vi "ExternalVIDefaultLoad.vi"(11 "VI in":refnum<vi>) -> (3 "Update?":bool)   [LabVIEW 2020]
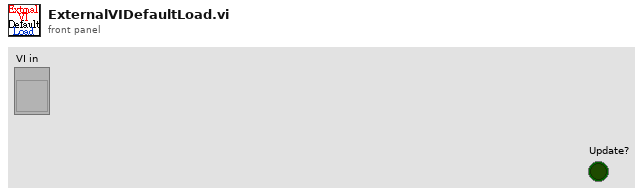
[diagram p1: front panel]
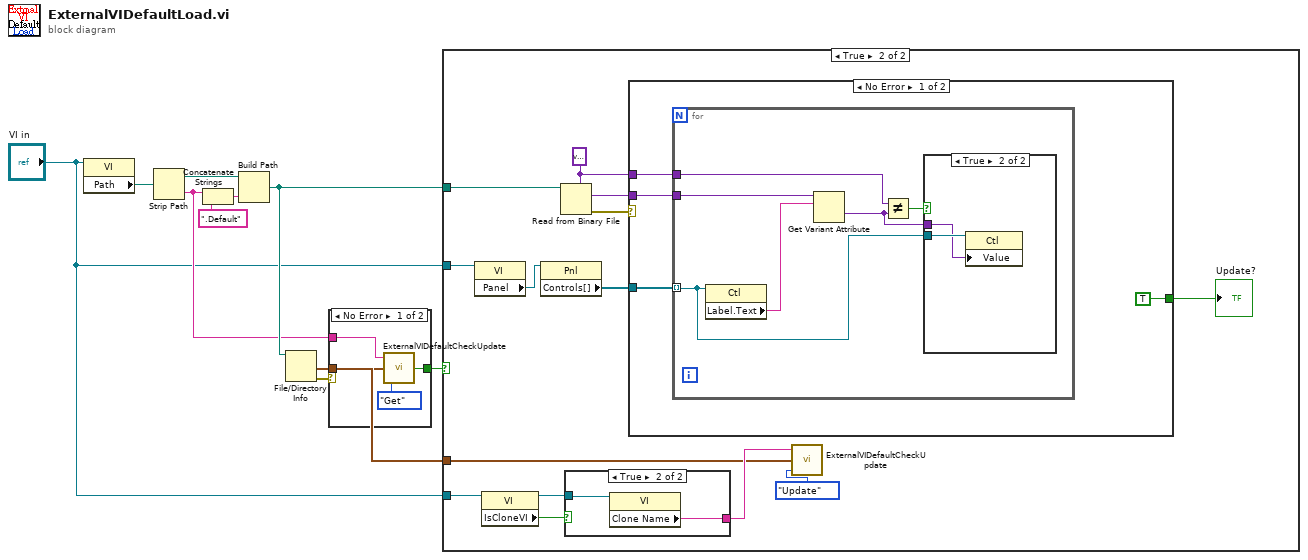
[diagram p0: block diagram]
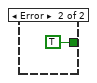
[diagram p2: hidden frame]
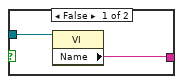
[diagram p4: hidden frame]
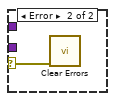
[diagram p6: hidden frame]
diagram:
  n1 = property class="VI"(reference="VI in") -> ("Path"=w7:path)  [unwired: 1 in, 2 out]
  n2 = Strip Path(path=w7) -> (stripped path=w9:path, name=w5:string)
  n3 = Concatenate Strings(w5, ".Default" ("string")) -> (w10:string)
  n4 = Build Path(base path=w9, name or relative path=w10) -> (appended path=w6:path)
  n5 = File/Directory Info(path=w6) -> (last mod=w3:timestamp, error out=w1:errorcluster)  [unwired: 1 in, 5 out]
  n6 = case shown="No Error" w1 {
    tunnel: w5 -> [w14 _]
    tunnel: [w12 TRUE ("NeedUpdate?")] -> w4
    tunnel: w3 -> [w11 _]
    frame No Error {
      n7 = call "ExternalVIDefaultCheckUpdate.vi"("OP"=enum16{"Get", "Update", "Init"}."Get", "last mod"=w11, "VIName"=w14) -> ("NeedUpdate?"=w12:bool)  [unwired: 1 in, 1 out]
    }
    frame Error {
    }
  }
  n8 = case shown="True" w4 {
    tunnel: "VI in" -> [_ w29]
    tunnel: w6 -> [_ w22]
    tunnel: w3 -> [_ w16]
    tunnel: "VI in" -> [_ w20]
    frame False {
    }
    frame True {
      w25 = variant
      n9 = property class="VI"(reference=w29) -> ("Panel"=w28:refnum<vi>)  [unwired: 1 in, 2 out]
      n10 = property class="VI"(reference=w20) -> (reference out=w18:refnum<vi>, "IsCloneVI"=w19:bool)  [unwired: 1 in, 1 out]
      n11 = property class="Pnl"(reference=w28) -> ("Controls[]"=w26:refnum<vi>[])  [unwired: 1 in, 2 out]
      n12 = Read from Binary File(5:w25, 11:w22) -> (0:w24:errorcluster, 2:w27:variant)  [unwired: 4 in, 2 out]
      n13 = case shown="True" w19 {
        tunnel: w18 -> [w31 w33]
        tunnel: [w30 w32] -> w17
        frame False {
          n14 = property class="VI"(reference=w31) -> ("Name"=w30:string)  [unwired: 1 in, 2 out]
        }
        frame True {
          n15 = property class="VI"(reference=w33) -> ("Clone Name"=w32:string)  [unwired: 1 in, 2 out]
        }
      }
      n16 = case shown="No Error" w24 {
        selector: w24 -> [_ w46]
        tunnel: w27 -> [w37 _]
        tunnel: w26 -> [w36 _]
        tunnel: w25 -> [w35 _]
        tunnel: [TRUE _] -> w23
        frame No Error {
          n17 = for {
            tunnel: w37 -> [w43]
            tunnel: w36 -> [w40] mode=indexing
            tunnel: w35 -> [w38]
            n18 = property class="Ctl"(reference=w40) -> ("Label.Text"=w42:string)  [unwired: 1 in, 2 out]
            n19 = Get Variant Attribute(Variant=w43, name=w42) -> (value=w39:variant)  [unwired: 2 in, 3 out]
            n20 = Not Equal?(x=w38, y=w39) -> (x != y?=w41:bool)
            n21 = case shown="True" w41 {
              tunnel: w40 -> [_ w45]
              tunnel: w39 -> [_ w44]
              frame False {
              }
              frame True {
                n22 = property class="Ctl"(reference=w45, "Value"=w44) -> ()  [unwired: 1 in, 2 out]
              }
            }
          }
        }
        frame Error {
          n23 = call <vilib>:"Clear Errors.vi"("error in (no error)"=w46) -> ()  [unwired: 5 in, 2 out]
        }
      }
      "Update?" <- w23
      n24 = call "ExternalVIDefaultCheckUpdate.vi"("OP"=enum16{"Get", "Update", "Init"}."Update", "last mod"=w16, "VIName"=w17) -> ()  [unwired: 1 in, 2 out]
    }
  }
